vi "Get Joystick 1 All.vi"(8 "error in (no error)":errorcluster) -> (0 "error out":errorcluster, 2 "Axes":dbl[](array[numeric]), 3 "Buttons":bool[](array[boolean]))   [LabVIEW 2014]
uses:
  <vilib>/Rock Robotics/WPI/Joystick/WPI_JoystickGetSetRefNum.vi
  <vilib>/Rock Robotics/Network Tables/SD Write Boolean Array.vi
  <vilib>/Rock Robotics/Network Tables/SD Write Numeric Array.vi
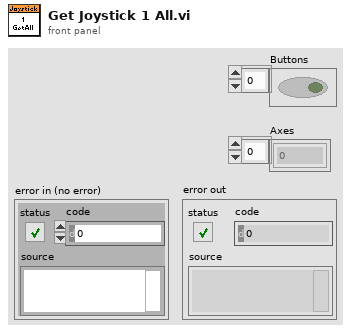
[diagram p1: front panel]
types:
  T1 = typedef "WPI_JoystickDevRef.ctl" = cluster{"Device":T2}
  T2 = typedef "WPI_JoystickDeviceEnum.ctl" = enum16{"USB 0", "USB 1", "USB 2", "USB 3", "USB 4", "USB 5"}
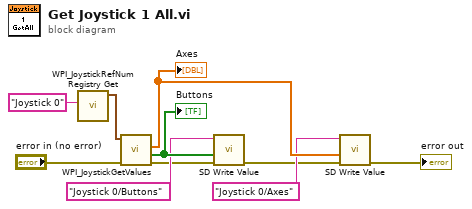
[diagram p0: block diagram]
diagram:
  n1 = call <vilib>:"WPI_JoystickRefNum Registry Get.vi"("refnum name"="Joystick 0") -> ("JoystickDevRef"=w8:T1)  [unwired: 9 in, 1 out]
  n2 = call <vilib>:"WPI_JoystickGetValues.vi"("error in (no error)"="error in (no error)", "JoystickDevRef"=w8) -> ("error out"=w3:errorcluster, "Buttons"=w10:bool[], "Axes"=w9:dbl[])  [unwired: 5 in, 2 out]
  "Buttons" <- w10
  "Axes" <- w9
  n3 = call-poly <vilib>:"SD Write Value.vi"("error in"=w3, "Boolean Array"=w10, "Name"="Joystick 0/Buttons") -> ("error out"=w2:errorcluster)  [unwired: 7 in, 1 out]
  n4 = call-poly <vilib>:"SD Write Value.vi"("error in"=w2, "Numeric Array"=w9, "Name"="Joystick 0/Axes") -> ("error out"=→"error out":errorcluster)  [unwired: 7 in, 1 out]
